vi "View.vi"(8 "error in (no error)":errorcluster, 11 "Laser View in":refnum<class "Laser View.lvclass">) -> (0 "error out":errorcluster, 3 "Laser View out":refnum<class "Laser View.lvclass">)   [LabVIEW 2022 SP3, in "Laser View.lvclass"]
uses:
  Laser View.lvclass
  C:/XY Stage/iView/base view/base view.lvclass
  Laser State Data/Laser State.ctl
  iView/base view/Accessors/Read View Refnum.vi
  iView/base view/base view.lvclass
  Laser Controller/Laser Controller.lvclass
  Laser View.lvclass/Laser View.ctl
  Laser State Data/Laser State Data.lvclass
panel:
  out "error out 2":errorcluster
  out "Laser Temp":cluster{" time":timestamp, "Temp":dbl}[](graph)
  out "Current Temp(C)":dbl
  out "Current Power":dbl
  out "Laser State":T1
  in  "Warm Laser":bool
  in  "Stop Laser":bool
  in  "Fire Laser":bool
  in  "Laser Power":dbl
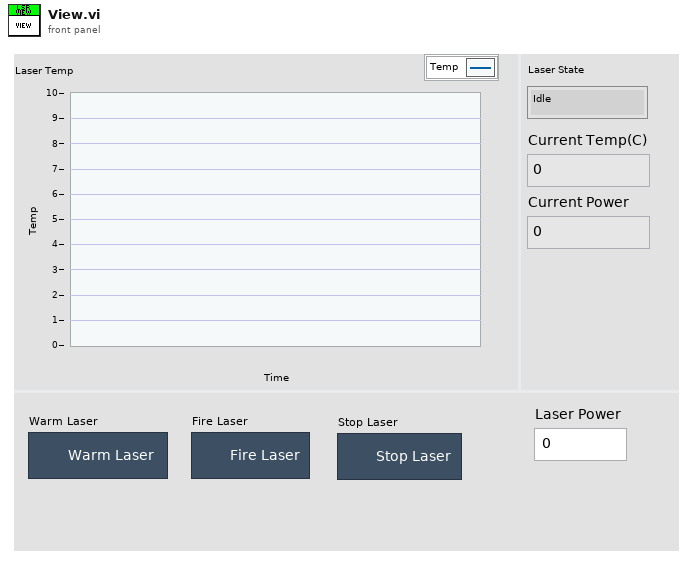
[diagram p1: front panel]
types:
  T1 = typedef "Laser State Data.lvclass/Laser State.ctl" = enum16{"Idle", "Warming", "Ready", "Firing"}
  T2 = typedef "base view.lvclass/Events.ctl" = cluster{"Open":refnum<user-event>, "Close":refnum<user-event>, "Hide":refnum<user-event>}
  T3 = cluster{"Laser State":refnum<event-registration>, "Laser Process State":refnum<event-registration>, "Event Registration Refnum":refnum<event-registration>}
  T4 = enum8{"Enabled", "Disabled", "Disabled and Grayed Out"}
  T5 = typedef "Laser State Data.lvclass/Time and Temp.ctl" = cluster{" time":timestamp, "Temp":dbl}
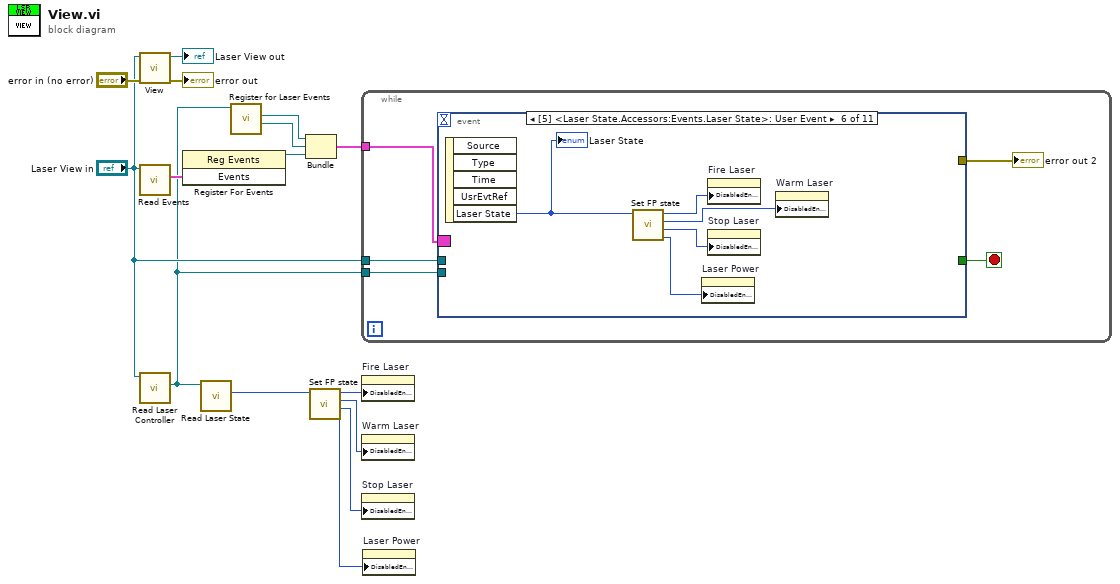
[diagram p0: block diagram]
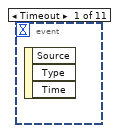
[diagram p2: hidden frame]
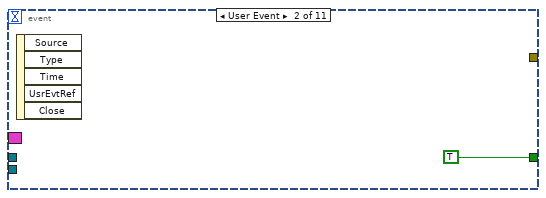
[diagram p3: hidden frame]
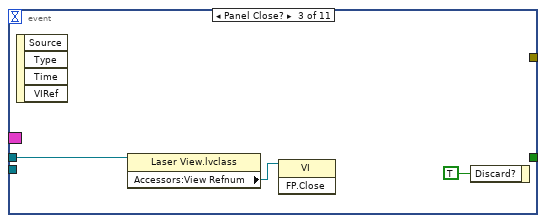
[diagram p4: hidden frame]
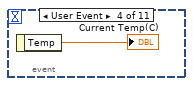
[diagram p5: hidden frame]
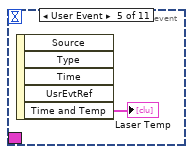
[diagram p6: hidden frame]
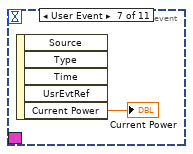
[diagram p7: hidden frame]
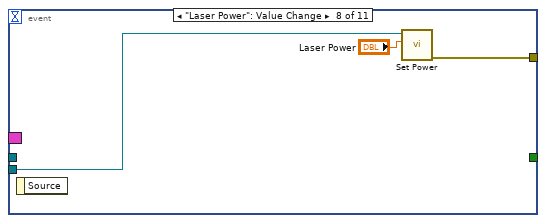
[diagram p8: hidden frame]
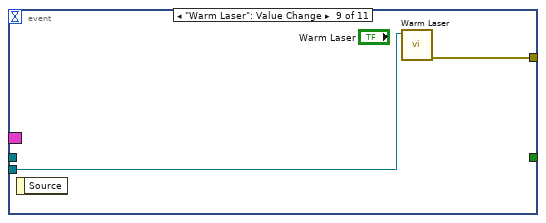
[diagram p9: hidden frame]
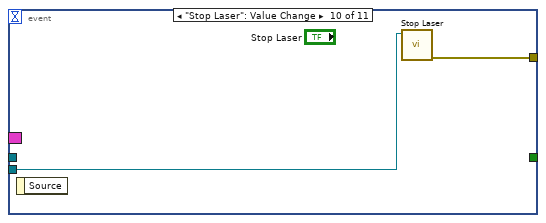
[diagram p10: hidden frame]
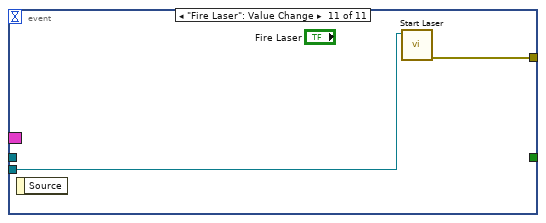
[diagram p11: hidden frame]
diagram:
  n1 = call-parent "View.vi"("error in (no error)"="error in (no error)", "base view in"="Laser View in") -> ("error out"=→"error out":errorcluster, "base view out"=→"Laser View out":refnum<class "Laser View.lvclass">)  [unwired: 8 in]
  n2 = call "Read Events.vi"("In"="Laser View in") -> ("Events"=w12:T2)  [unwired: 8 in, 2 out]
  n3 = call "Read Laser Controller.vi"("In"="Laser View in") -> ("Laser Controller"=w6:refnum<class "Laser Controller.lvclass">)  [unwired: 8 in, 2 out]
  n4 = register-events(w12) -> (reference out=w9:refnum<event-registration>)  [unwired: 2 in, 1 out]
  n5 = call-dynamic "Read Laser State.vi"("Laser Controller in"=w6) -> ("Laser State"=w5:T1)  [unwired: 8 in, 2 out]
  n6 = call-dynamic "Register for Laser Events.vi"("Laser Controller in"=w6) -> ("Laser Process State"=w10:refnum<event-registration>, "Laser State"=w11:refnum<event-registration>)  [unwired: 7 in, 2 out]
  n7 = Bundle("Laser State"=w11, "Laser Process State"=w10, "Event Registration Refnum"=w9) -> (w8:T3)  [unwired: 1 in]
  n8 = call "Set FP state.vi"("Laser State"=w5) -> ("Laser Power"=w1:T4, "stop laser"=w2:T4, "warm laser"=w3:T4, "Fire laser"=w4:T4)  [unwired: 7 in]
  n9 = while {
    tunnel: w8 -> [w20]
    tunnel: "Laser View in" -> [w18]
    tunnel: w6 -> [w17]
    stop <- w19 stop-if-true
    n10 = event shown="[5] <Laser State.Accessors:Events.Laser State>: User Event" {
      selector: w20 -> [_ _ _ _ _ _ _ _ _ _ _]
      dyn-events: _ -> [_ _ _ _ _ _ _ _ _ _ _]
      timeout: _ -> [_ _ _ _ _ _ _ _ _ _ _]
      tunnel: [_ TRUE _ _ _ _ _ _ _ _ _] -> w19
      tunnel: w18 -> [_ _ w23 _ _ _ _ _ _ _ _]
      tunnel: w17 -> [_ _ _ _ _ _ _ w35 w37 w39 w41]
      tunnel: [_ _ _ _ _ _ _ w33 w36 w38 w40] -> w16
      event Timeout {
        n11 = event-data() -> ()  [unwired: 1 in, 3 out]
      }
      event User Event {
        n12 = event-data() -> ()  [unwired: 1 in, 5 out]
      }
      event Panel Close? {
        n13 = event-data() -> ()  [unwired: 1 in, 4 out]
        n14 = property class="Laser View.lvclass"(reference=w23) -> ("Accessors:View Refnum"=w24:refnum<vi>)  [unwired: 1 in, 2 out]
        n15 = invoke class="VI" method="FP.Close"(reference=w24) -> ()  [unwired: 2 in, 3 out]
        n16 = event-data("Discard?"=TRUE) -> ()  [unwired: 1 in, 1 out]
      }
      event User Event {
        n17 = event-data() -> ("Temp"=→"Current Temp(C)":dbl)  [unwired: 1 in]
      }
      event User Event {
        n18 = event-data() -> ("Time and Temp"=→"Laser Temp":T5[])  [unwired: 1 in, 4 out]
      }
      event User Event {
        n19 = event-data() -> ("Laser State"=w31:T1)  [unwired: 1 in, 4 out]
        "Laser State" <- w31
        n20 = call "Set FP state.vi"("Laser State"=w31) -> ("Laser Power"=w27:T4, "stop laser"=w29:T4, "warm laser"=w30:T4, "Fire laser"=w28:T4)  [unwired: 7 in]
        n21 = property on="Laser Power" class="DigNum (strict)"("DisabledEnum"=w27) -> ()  [unwired: 2 in, 2 out]
        n22 = property on="Fire Laser" class="Bool"("DisabledEnum"=w28) -> ()  [unwired: 2 in, 2 out]
        n23 = property on="Stop Laser" class="Bool"("DisabledEnum"=w29) -> ()  [unwired: 2 in, 2 out]
        n24 = property on="Warm Laser" class="Bool"("DisabledEnum"=w30) -> ()  [unwired: 2 in, 2 out]
      }
      event User Event {
        n25 = event-data() -> ("Current Power"=→"Current Power":dbl)  [unwired: 1 in, 4 out]
      }
      event "Laser Power": Value Change {
        n26 = event-data() -> ()  [unwired: 1 in, 1 out]
        n27 = call-dynamic "Set Power.vi"("Power"="Laser Power", "Laser Controller API in"=w35) -> ("error out"=w33:errorcluster)  [unwired: 8 in, 1 out]
      }
      event "Warm Laser": Value Change {
        n28 = event-data() -> ()  [unwired: 1 in, 1 out]
        n29 = call-dynamic "Warm Laser.vi"("Laser Controller API in"=w37) -> ("error out"=w36:errorcluster)  [unwired: 9 in, 1 out]
      }
      event "Stop Laser": Value Change {
        n30 = event-data() -> ()  [unwired: 1 in, 1 out]
        n31 = call-dynamic "Stop Laser.vi"("Laser Controller API in"=w39) -> ("error out"=w38:errorcluster)  [unwired: 9 in, 1 out]
      }
      event "Fire Laser": Value Change {
        n32 = event-data() -> ()  [unwired: 1 in, 1 out]
        n33 = call-dynamic "Start Laser.vi"("Laser Controller API in"=w41) -> ("error out"=w40:errorcluster)  [unwired: 9 in, 1 out]
      }
    }
    "error out 2" <- w16
  }
  n34 = property on="Fire Laser" class="Bool"("DisabledEnum"=w4) -> ()  [unwired: 2 in, 2 out]
  n35 = property on="Warm Laser" class="Bool"("DisabledEnum"=w3) -> ()  [unwired: 2 in, 2 out]
  n36 = property on="Stop Laser" class="Bool"("DisabledEnum"=w2) -> ()  [unwired: 2 in, 2 out]
  n37 = property on="Laser Power" class="DigNum (strict)"("DisabledEnum"=w1) -> ()  [unwired: 2 in, 2 out]
